vi "Generate_Raster_V8_Daq6363_CtrBased.vi"(0 "X Parameters":T3={"Number of Steps"=500, "Max X"=2.0, "Min X"=-2.0}, 1 "Scan Pattern":T2(ring)=enum."1x B-scan", 3 "X Offset":dbl, 5 "Y Parameters":T4={"Number of Steps"=500, "Max Y"=2.0, "Min Y"=-2.0}, 9 "Camera Param":T1={"B-scan Period"=0.0, "Return Time"=1.0, "Scan Rate"=40.0, "Duty Cycle"=0.95, "Camera Delay"=0.0}, 11 "error in (no error)":errorcluster, 12 "angle":dbl, 14 "Y Offset":dbl) -> (6 "Galvo Array":dbl[][](array[numeric]), 15 "error IO":errorcluster)   [LabVIEW 2019]
panel:
  out "size(s)":i32=270000
  out "Galvo Array 2":dbl[][](graph)
  # "AO1: X Galvo"
  # "AO0: Y Galvo"
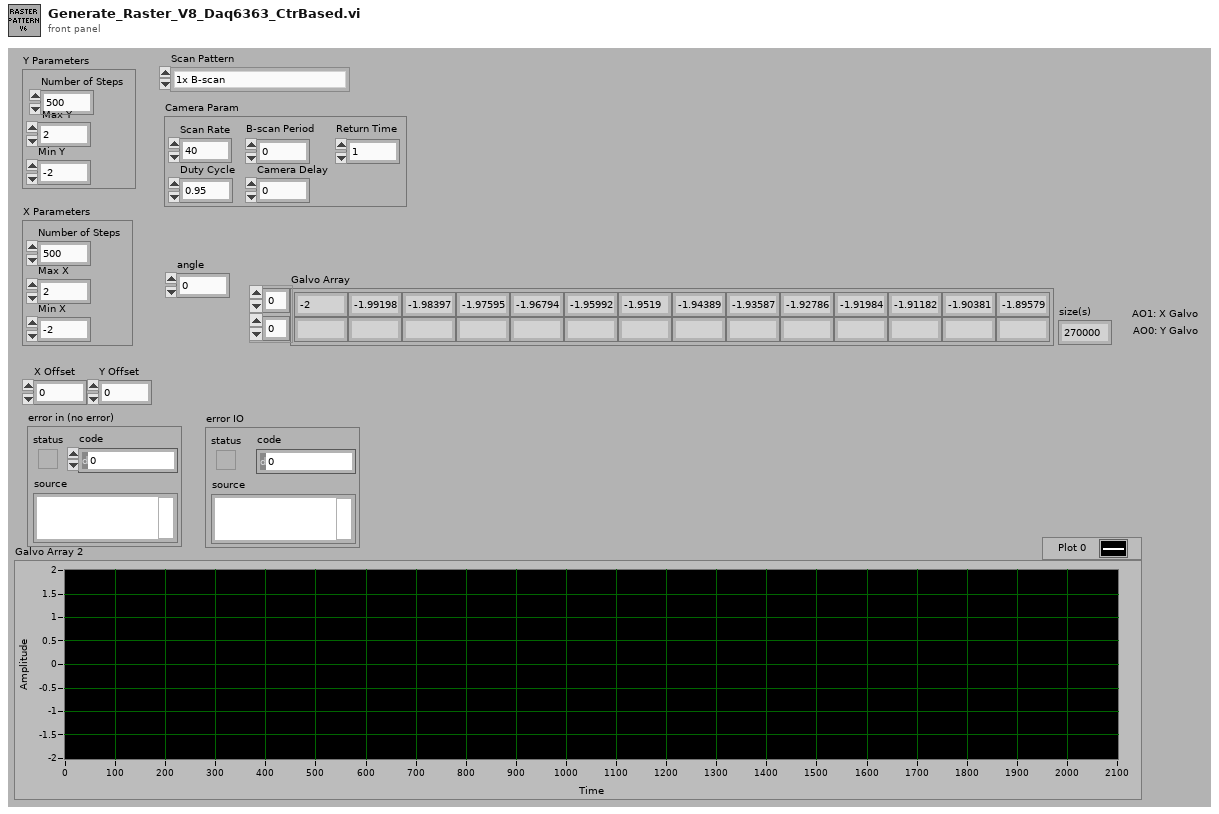
[diagram p1: front panel]
types:
  T1 = cluster{"B-scan Period":dbl, "Return Time":dbl, "Scan Rate":dbl, "Duty Cycle":dbl, "Camera Delay":dbl}
  T2 = enum16{"2D Uni Dir", "2D Bi Dir", "1x B-scan", "2x B-scan", "3x B-scan", "4x B-scan", "5x B-scan", "10x B-scan", "1x B-scan (Bi-Directional)", "2x B-scan (Bi-Directional)", "5x B-scan (Bi-Directional)", "10x B-scan (Bi-Directional)"}
  T3 = cluster{"Number of Steps":i32, "Max X":dbl, "Min X":dbl}
  T4 = cluster{"Number of Steps":i32, "Max Y":dbl, "Min Y":dbl}
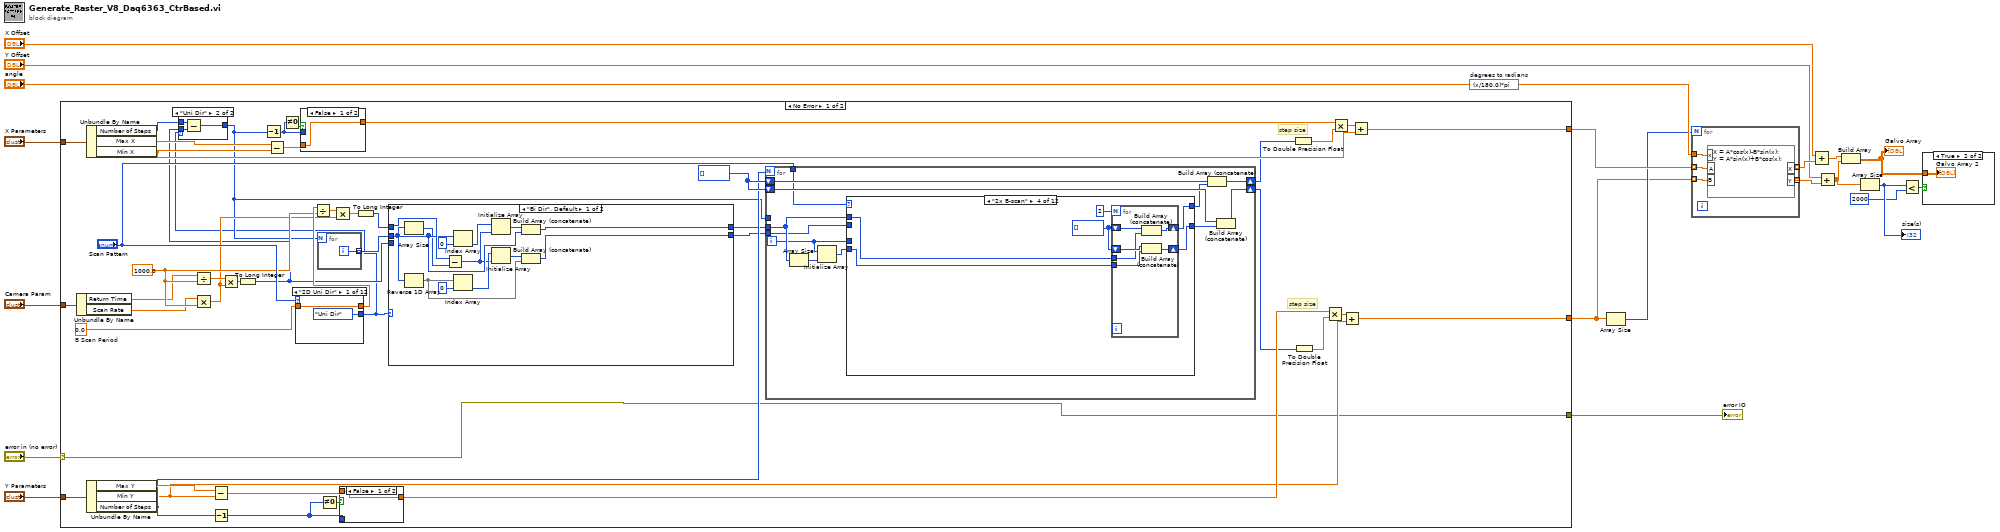
[diagram p0: block diagram]
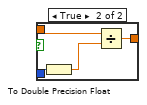
[diagram p4: hidden frame]
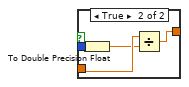
[diagram p5: hidden frame]
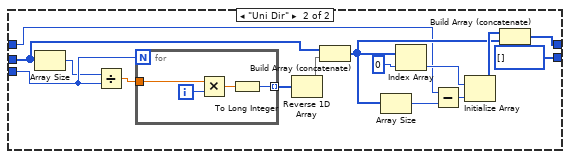
[diagram p6: hidden frame]
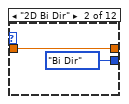
[diagram p7: hidden frame]
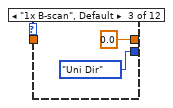
[diagram p8: hidden frame]
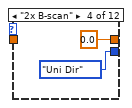
[diagram p9: hidden frame]
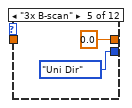
[diagram p10: hidden frame]
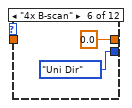
[diagram p11: hidden frame]
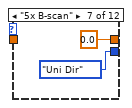
[diagram p12: hidden frame]
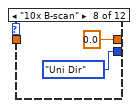
[diagram p13: hidden frame]
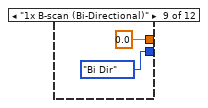
[diagram p14: hidden frame]
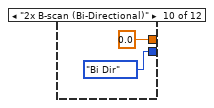
[diagram p15: hidden frame]
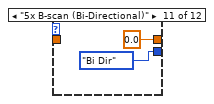
[diagram p16: hidden frame]
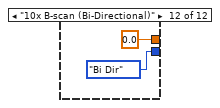
[diagram p17: hidden frame]
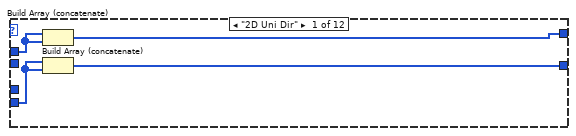
[diagram p18: hidden frame]
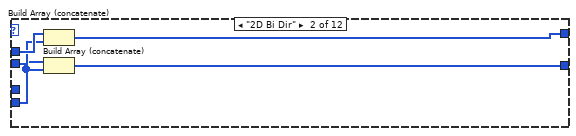
[diagram p19: hidden frame]
diagram:
  n1 = case shown="No Error" "error in (no error)" {
    selector: "error in (no error)" -> [w24 w337]
    tunnel: "X Parameters" -> [w65 _]
    tunnel: "Y Parameters" -> [w64 _]
    tunnel: [w24 w337] -> w20
    tunnel: [w47 w336] -> w14
    tunnel: [w36 w336] -> w9
    tunnel: "Camera Param" -> [w23 _]
    frame No Error {
      w25 = 0.0  # B Scan Period
      w35 = 1000.0 ("y")
      w58 = i32[] []
      # "step size"
      # "step size"
      n2 = Unbundle By Name(w23) -> ("Return Time"=w22:dbl, "Scan Rate"=w21:dbl)
      n3 = Unbundle By Name(w65) -> ("Number of Steps"=w28:i32, "Max X"=w62:dbl, "Min X"=w56:dbl)
      n4 = Unbundle By Name(w64) -> ("Max Y"=w63:dbl, "Min Y"=w37:dbl, "Number of Steps"=w55:i32)
      n5 = Divide(x=w22, y=w35) -> (x/y=w52:dbl)
      n6 = Multiply(x=w21, y=w35) -> (x*y=w34:dbl)
      n7 = Subtract(x=w63, y=w37) -> (x-y=w61:dbl)
      n8 = Decrement(x=w55) -> (x-1=w30:i32)
      n9 = Multiply(x=w52, y=w34) -> (x*y=w51:dbl)
      n10 = To Long Integer(number=w51) -> (32bit integer=w27:i32)
      n11 = Subtract(x=w62, y=w56) -> (x-y=w57:dbl)
      n12 = case shown="\"2D Uni Dir\"" "Scan Pattern" {
        tunnel: [enum16{"Bi Dir", "Uni Dir"}."Uni Dir" enum16{"Bi Dir", "Uni Dir"}."Bi Dir" enum16{"Bi Dir", "Uni Dir"}."Uni Dir" enum16{"Bi Dir", "Uni Dir"}."Uni Dir" enum16{"Bi Dir", "Uni Dir"}."Uni Dir" enum16{"Bi Dir", "Uni Dir"}."Uni Dir" enum16{"Bi Dir", "Uni Dir"}."Uni Dir" enum16{"Bi Dir", "Uni Dir"}."Uni Dir" enum16{"Bi Dir", "Uni Dir"}."Bi Dir" enum16{"Bi Dir", "Uni Dir"}."Bi Dir" enum16{"Bi Dir", "Uni Dir"}."Bi Dir" enum16{"Bi Dir", "Uni Dir"}."Bi Dir"] -> w26
        tunnel: w25 -> [w113 w116 _ _ _ _ _ _ _ _ _ _]
        tunnel: [w113 w116 0.0 ("B-scan Period") 0.0 ("B-scan Period") 0.0 ("B-scan Period") 0.0 ("B-scan Period") 0.0 ("B-scan Period") 0.0 ("B-scan Period") 0.0 ("B-scan Period") 0.0 ("B-scan Period") 0.0 ("B-scan Period") 0.0 ("B-scan Period")] -> w45
        frame "2D Uni Dir" {
        }
        frame "2D Bi Dir" {
        }
        frame "1x B-scan", Default {
        }
        frame "2x B-scan" {
        }
        frame "3x B-scan" {
        }
        frame "4x B-scan" {
        }
        frame "5x B-scan" {
        }
        frame "10x B-scan" {
        }
        frame "1x B-scan (Bi-Directional)" {
        }
        frame "2x B-scan (Bi-Directional)" {
        }
        frame "5x B-scan (Bi-Directional)" {
        }
        frame "10x B-scan (Bi-Directional)" {
        }
      }
      n13 = case shown="\"Uni Dir\"" w26 {
        tunnel: [w66 w69] -> w29
        tunnel: w28 -> [w66 w68]
        tunnel: w27 -> [_ w67]
        frame "Bi Dir", Default {
        }
        frame "Uni Dir" {
          n14 = Subtract(x=w68, y=w67) -> (x-y=w69:i32)
        }
      }
      n15 = Decrement(x=w29) -> (x-1=w32:i32)
      n16 = Not Equal To 0?(x=w32) -> (x != 0?=w33:bool)
      n17 = case shown="False" w33 {
        tunnel: w57 -> [w75 w79]
        tunnel: w32 -> [_ w77]
        tunnel: [w75 w76] -> w40
        frame False {
        }
        frame True {
          n18 = To Double Precision Float(number=w77) -> (double precision float=w78:dbl)
          n19 = Divide(x=w79, y=w78) -> (x/y=w76:dbl)
        }
      }
      n20 = Divide(x=w45, y=w35) -> (x/y=w54:dbl)
      n21 = for {
        N: w29 -> [_]
        tunnel: [w112] -> w43 mode=indexing
        i -> [w112]
      }
      n22 = Not Equal To 0?(x=w30) -> (x != 0?=w31:bool)
      n23 = Multiply(x=w54, y=w34) -> (x*y=w53:dbl)
      n24 = case shown="False" w31 {
        tunnel: w61 -> [w70 w74]
        tunnel: [w70 w72] -> w59
        tunnel: w30 -> [_ w71]
        frame False {
        }
        frame True {
          n25 = To Double Precision Float(number=w71) -> (double precision float=w73:dbl)
          n26 = Divide(x=w74, y=w73) -> (x/y=w72:dbl)
        }
      }
      n27 = To Long Integer(number=w53) -> (32bit integer=w44:i32)
      n28 = case shown="\"Bi Dir\", Default" w26 {
        tunnel: w43 -> [w88 w100]
        tunnel: [w83 w97] -> w42
        tunnel: w44 -> [w92 w99]
        tunnel: w27 -> [_ w98]
        tunnel: [w82 i32[] []] -> w41
        frame "Bi Dir", Default {
          n29 = Array Size(array=w88) -> (size(s)=w81:i32)
          n30 = Reverse 1D Array(array=w88) -> (reversed array=w84:i32[])
          n31 = Subtract(x=w92, y=w81) -> (x-y=w80:i32)
          n32 = Index Array(array=w88, index=0) -> (element=w91:i32)
          n33 = Index Array(array=w84, index=0) -> (element=w87:i32)
          n34 = Initialize Array(w91, w80) -> (w89:i32[])
          n35 = Initialize Array(w87, w80) -> (w85:i32[])
          n36 = Build Array (concatenate)(w89, w88) -> (w83:i32[])
          n37 = Build Array (concatenate)(w85, w84) -> (w82:i32[])
        }
        frame "Uni Dir" {
          n38 = Array Size(array=w100) -> (size(s)=w95:i32)
          n39 = Divide(x=w95, y=w98) -> (x/y=w104:dbl)
          n40 = for {
            N: w98 -> [_]
            tunnel: w104 -> [w110]
            tunnel: [w108] -> w107 mode=indexing
            i -> [w111]
            n41 = Multiply(x=w110, y=w111) -> (x*y=w109:dbl)
            n42 = To Long Integer(number=w109) -> (32bit integer=w108:i32)
          }
          n43 = Reverse 1D Array(array=w107) -> (reversed array=w106:i32[])
          n44 = Build Array (concatenate)(w100, w106) -> (w101:i32[])
          n45 = Array Size(array=w101) -> (size(s)=w94:i32)
          n46 = Index Array(array=w101, index=0) -> (element=w105:i32)
          n47 = Subtract(x=w99, y=w94) -> (x-y=w93:i32)
          n48 = Initialize Array(w105, w93) -> (w102:i32[])
          n49 = Build Array (concatenate)(w102, w101) -> (w97:i32[])
        }
      }
      n50 = for {
        N: w55 -> [_]
        shift-right: [w147] -> w49
        shift-left: w58 -> [w145]
        shift-right: [w148] -> w50
        shift-left: w58 -> [w146]
        tunnel: w29 -> [_]
        tunnel: "Scan Pattern" -> [w144]
        tunnel: w42 -> [w142]
        tunnel: w41 -> [w140]
        i -> [w137]
        n51 = Array Size(array=w142) -> (size(s)=w141:i32)
        n52 = Initialize Array(w137, w141) -> (w143:i32[])
        n53 = case shown="\"2x B-scan\"" w144 {
          tunnel: [w149 w155 w158 w160 w172 w184 w196 w209 w221 w250 w279 w308] -> w139
          tunnel: [w151 w153 w159 w161 w173 w185 w197 w210 w222 w251 w280 w309] -> w138
          tunnel: w143 -> [w152 w154 w159 w164 w176 w188 w200 w213 w225 w254 w283 w312]
          tunnel: w142 -> [w150 w157 w158 w163 w175 w187 w199 w212 w224 w253 w282 w311]
          tunnel: w137 -> [_ _ _ _ _ _ _ _ w220 w249 w278 w307]
          tunnel: w140 -> [_ w156 _ _ _ _ _ _ w223 w252 w281 w310]
          frame "2D Uni Dir" {
            n54 = Build Array (concatenate)(w150, w150) -> (w149:i32[])
            n55 = Build Array (concatenate)(w152, w152) -> (w151:i32[])
          }
          frame "2D Bi Dir" {
            n56 = Build Array (concatenate)(w157, w156) -> (w155:i32[])
            n57 = Build Array (concatenate)(w154, w154) -> (w153:i32[])
          }
          frame "1x B-scan", Default {
          }
          frame "2x B-scan" {
            w162 = i32[] []
            n58 = for {
              N: 2 -> [_]
              shift-right: [w170] -> w161
              shift-left: w162 -> [w171]
              tunnel: w164 -> [w169]
              shift-right: [w168] -> w160
              shift-left: w162 -> [w167]
              tunnel: w163 -> [w166]
              n59 = Build Array (concatenate)(w167, w166) -> (w168:i32[])
              n60 = Build Array (concatenate)(w171, w169) -> (w170:i32[])
            }
          }
          frame "3x B-scan" {
            w174 = i32[] []
            n61 = for {
              N: 3 -> [_]
              shift-right: [w182] -> w173
              shift-left: w174 -> [w183]
              tunnel: w176 -> [w181]
              shift-right: [w180] -> w172
              shift-left: w174 -> [w179]
              tunnel: w175 -> [w178]
              n62 = Build Array (concatenate)(w179, w178) -> (w180:i32[])
              n63 = Build Array (concatenate)(w183, w181) -> (w182:i32[])
            }
          }
          frame "4x B-scan" {
            w186 = i32[] []
            n64 = for {
              N: 4 -> [_]
              shift-right: [w194] -> w185
              shift-left: w186 -> [w195]
              tunnel: w188 -> [w193]
              shift-right: [w192] -> w184
              shift-left: w186 -> [w191]
              tunnel: w187 -> [w190]
              n65 = Build Array (concatenate)(w191, w190) -> (w192:i32[])
              n66 = Build Array (concatenate)(w195, w193) -> (w194:i32[])
            }
          }
          frame "5x B-scan" {
            w198 = i32[] []
            n67 = for {
              N: 5 -> [_]
              shift-right: [w206] -> w197
              shift-left: w198 -> [w207]
              tunnel: w200 -> [w205]
              shift-right: [w204] -> w196
              shift-left: w198 -> [w203]
              tunnel: w199 -> [w202]
              n68 = Build Array (concatenate)(w203, w202) -> (w204:i32[])
              n69 = Build Array (concatenate)(w207, w205) -> (w206:i32[])
            }
          }
          frame "10x B-scan" {
            w211 = i32[] []
            n70 = for {
              N: 10 -> [_]
              shift-right: [w218] -> w210
              shift-left: w211 -> [w219]
              tunnel: w213 -> [w217]
              shift-right: [w216] -> w209
              shift-left: w211 -> [w215]
              tunnel: w212 -> [w214]
              n71 = Build Array (concatenate)(w215, w214) -> (w216:i32[])
              n72 = Build Array (concatenate)(w219, w217) -> (w218:i32[])
            }
          }
          frame "1x B-scan (Bi-Directional)" {
            w226 = i32[] []
            n73 = for {
              N: 1 -> [w232]
              shift-right: [w241] -> w222
              shift-left: w226 -> [w242]
              tunnel: w225 -> [w240]
              shift-right: [w239] -> w221
              shift-left: w226 -> [w238]
              tunnel: w224 -> [w237]
              tunnel: w223 -> [w233]
              tunnel: w220 -> [w231]
              i -> [w230]
              n74 = Multiply(x=w232, y=w231) -> (x*y=w229:i32)
              n75 = Build Array (concatenate)(w242, w240) -> (w241:i32[])
              n76 = Add(x=w229, y=w230) -> (x+y=w228:i32)
              n77 = Quotient & Remainder(x=w228, y=2) -> (x-y*floor(x/y)=w235:i32)  [unwired: 1 out]
              n78 = Equal To 0?(x=w235) -> (x = 0?=w234:bool)
              n79 = case shown="True" w234 {
                tunnel: [w243 w248] -> w239
                tunnel: w238 -> [w245 w247]
                tunnel: w237 -> [_ w246]
                tunnel: w233 -> [w244 _]
                frame False {
                  n80 = Build Array (concatenate)(w245, w244) -> (w243:i32[])
                }
                frame True {
                  n81 = Build Array (concatenate)(w247, w246) -> (w248:i32[])
                }
              }
            }
          }
          frame "2x B-scan (Bi-Directional)" {
            w255 = i32[] []
            n82 = for {
              N: 2 -> [w261]
              shift-right: [w270] -> w251
              shift-left: w255 -> [w271]
              tunnel: w254 -> [w269]
              shift-right: [w268] -> w250
              shift-left: w255 -> [w267]
              tunnel: w253 -> [w266]
              tunnel: w252 -> [w262]
              tunnel: w249 -> [w260]
              i -> [w259]
              n83 = Multiply(x=w261, y=w260) -> (x*y=w258:i32)
              n84 = Build Array (concatenate)(w271, w269) -> (w270:i32[])
              n85 = Add(x=w258, y=w259) -> (x+y=w257:i32)
              n86 = Quotient & Remainder(x=w257, y=2) -> (x-y*floor(x/y)=w264:i32)  [unwired: 1 out]
              n87 = Equal To 0?(x=w264) -> (x = 0?=w263:bool)
              n88 = case shown="False" w263 {
                tunnel: [w272 w277] -> w268
                tunnel: w267 -> [w274 w276]
                tunnel: w266 -> [_ w275]
                tunnel: w262 -> [w273 _]
                frame False {
                  n89 = Build Array (concatenate)(w274, w273) -> (w272:i32[])
                }
                frame True {
                  n90 = Build Array (concatenate)(w276, w275) -> (w277:i32[])
                }
              }
            }
          }
          frame "5x B-scan (Bi-Directional)" {
            w284 = i32[] []
            n91 = for {
              N: 5 -> [w290]
              shift-right: [w299] -> w280
              shift-left: w284 -> [w300]
              tunnel: w283 -> [w298]
              shift-right: [w297] -> w279
              shift-left: w284 -> [w296]
              tunnel: w282 -> [w295]
              tunnel: w281 -> [w291]
              tunnel: w278 -> [w289]
              i -> [w288]
              n92 = Multiply(x=w290, y=w289) -> (x*y=w287:i32)
              n93 = Build Array (concatenate)(w300, w298) -> (w299:i32[])
              n94 = Add(x=w287, y=w288) -> (x+y=w286:i32)
              n95 = Quotient & Remainder(x=w286, y=2) -> (x-y*floor(x/y)=w293:i32)  [unwired: 1 out]
              n96 = Equal To 0?(x=w293) -> (x = 0?=w292:bool)
              n97 = case shown="True" w292 {
                tunnel: [w301 w306] -> w297
                tunnel: w296 -> [w303 w305]
                tunnel: w295 -> [_ w304]
                tunnel: w291 -> [w302 _]
                frame False {
                  n98 = Build Array (concatenate)(w303, w302) -> (w301:i32[])
                }
                frame True {
                  n99 = Build Array (concatenate)(w305, w304) -> (w306:i32[])
                }
              }
            }
          }
          frame "10x B-scan (Bi-Directional)" {
            w313 = i32[] []
            n100 = for {
              N: 10 -> [w319]
              shift-right: [w328] -> w309
              shift-left: w313 -> [w329]
              tunnel: w312 -> [w327]
              shift-right: [w326] -> w308
              shift-left: w313 -> [w325]
              tunnel: w311 -> [w324]
              tunnel: w310 -> [w320]
              tunnel: w307 -> [w318]
              i -> [w317]
              n101 = Multiply(x=w319, y=w318) -> (x*y=w316:i32)
              n102 = Build Array (concatenate)(w329, w327) -> (w328:i32[])
              n103 = Add(x=w316, y=w317) -> (x+y=w315:i32)
              n104 = Quotient & Remainder(x=w315, y=2) -> (x-y*floor(x/y)=w322:i32)  [unwired: 1 out]
              n105 = Equal To 0?(x=w322) -> (x = 0?=w321:bool)
              n106 = case shown="True" w321 {
                tunnel: [w330 w335] -> w326
                tunnel: w325 -> [w332 w334]
                tunnel: w324 -> [_ w333]
                tunnel: w320 -> [w331 _]
                frame False {
                  n107 = Build Array (concatenate)(w332, w331) -> (w330:i32[])
                }
                frame True {
                  n108 = Build Array (concatenate)(w334, w333) -> (w335:i32[])
                }
              }
            }
          }
        }
        n109 = Build Array (concatenate)(w145, w139) -> (w147:i32[])
        n110 = Build Array (concatenate)(w146, w138) -> (w148:i32[])
      }
      n111 = To Double Precision Float(number=w49) -> (double precision float=w39:dbl[])
      n112 = To Double Precision Float(number=w50) -> (double precision float=w60:dbl[])
      n113 = Multiply(x=w59, y=w60) -> (x*y=w38:dbl[])
      n114 = Multiply(x=w40, y=w39) -> (x*y=w48:dbl[])
      n115 = Add(x=w38, y=w37) -> (x+y=w36:dbl[])
      n116 = Add(x=w48, y=w56) -> (x+y=w47:dbl[])
    }
    frame Error {
      w336 = dbl[] []
    }
  }
  "error IO" <- w20
  n117 = expression code="(x/180.0)*pi" "degrees to radians"("angle") -> (w15:dbl)
  n118 = Array Size(array=w9) -> (size(s)=w11:i32)
  n119 = for {
    N: w11 -> [_]
    tunnel: w14 -> [w342] mode=indexing
    tunnel: w15 -> [w341]
    tunnel: [w340] -> w13 mode=indexing
    tunnel: w9 -> [w339] mode=indexing
    tunnel: [w338] -> w8 mode=indexing
    n120 = formula code="X = A*cos(x)-B*sin(x);\nY = A*sin(x)+B*cos(x);"("x"=w341, "A"=w342, "B"=w339) -> ("X"=w340:dbl, "Y"=w338:dbl)
  }
  n121 = Add(x="X Offset", y=w13) -> (x+y=w12:dbl[])
  n122 = Add(x="Y Offset", y=w8) -> (x+y=w6:dbl[])
  n123 = Build Array(w12, w6) -> (w2:dbl[][])
  "Galvo Array" <- w2
  n124 = Array Size(array=w6) -> (size(s)=w5:i32)
  "size(s)" <- w5
  n125 = Less?(x=w5, y=2000) -> (x < y?=w3:bool)
  n126 = case shown="True" w3 {
    tunnel: w2 -> [_ w343]
    frame False {
    }
    frame True {
      "Galvo Array 2" <- w343
    }
  }
